vi "Untitled 4.vi"() -> ()   [LabVIEW 2021]
uses:
  <vilib>/userDefined/High Color/IMAQdx.ctl
  <vilib>/MakerHub/LINX/Public/Utilities/Open Serial.vi
  <vilib>/MakerHub/LINX/Public/Sensors/Motion/Servo/Servo Open One Channel.vi
  <vilib>/MakerHub/LINX/Public/Sensors/Motion/Servo/Servo Set Pulse Width One Channel.vi
  <vilib>/MakerHub/LINX/Public/Sensors/Motion/Servo/Servo Close One Channel.vi
  <vilib>/MakerHub/LINX/LMH-LINX.lvlib
  <vilib>/MakerHub/LINX/Public/Sensors/Motion/Servo/Servo.lvlib
  <vilib>/vision/driver/NI_Vision_Acquisition_Software.lvlib
  <vilib>/vision/NI_Vision_Development_Module.lvlib
panel:
  out "Red":bool
  out "Blue":bool
  out "Green":bool
  out "Color Spectrum":dbl[](array[numeric]) format="%.2f"
  out "Image":T1(plugin-control)
  in  "x .or. y?":bool
  out "Error Out":errorcluster
  in  "Serial Port":refnum<visa-resource-name>="N/A"
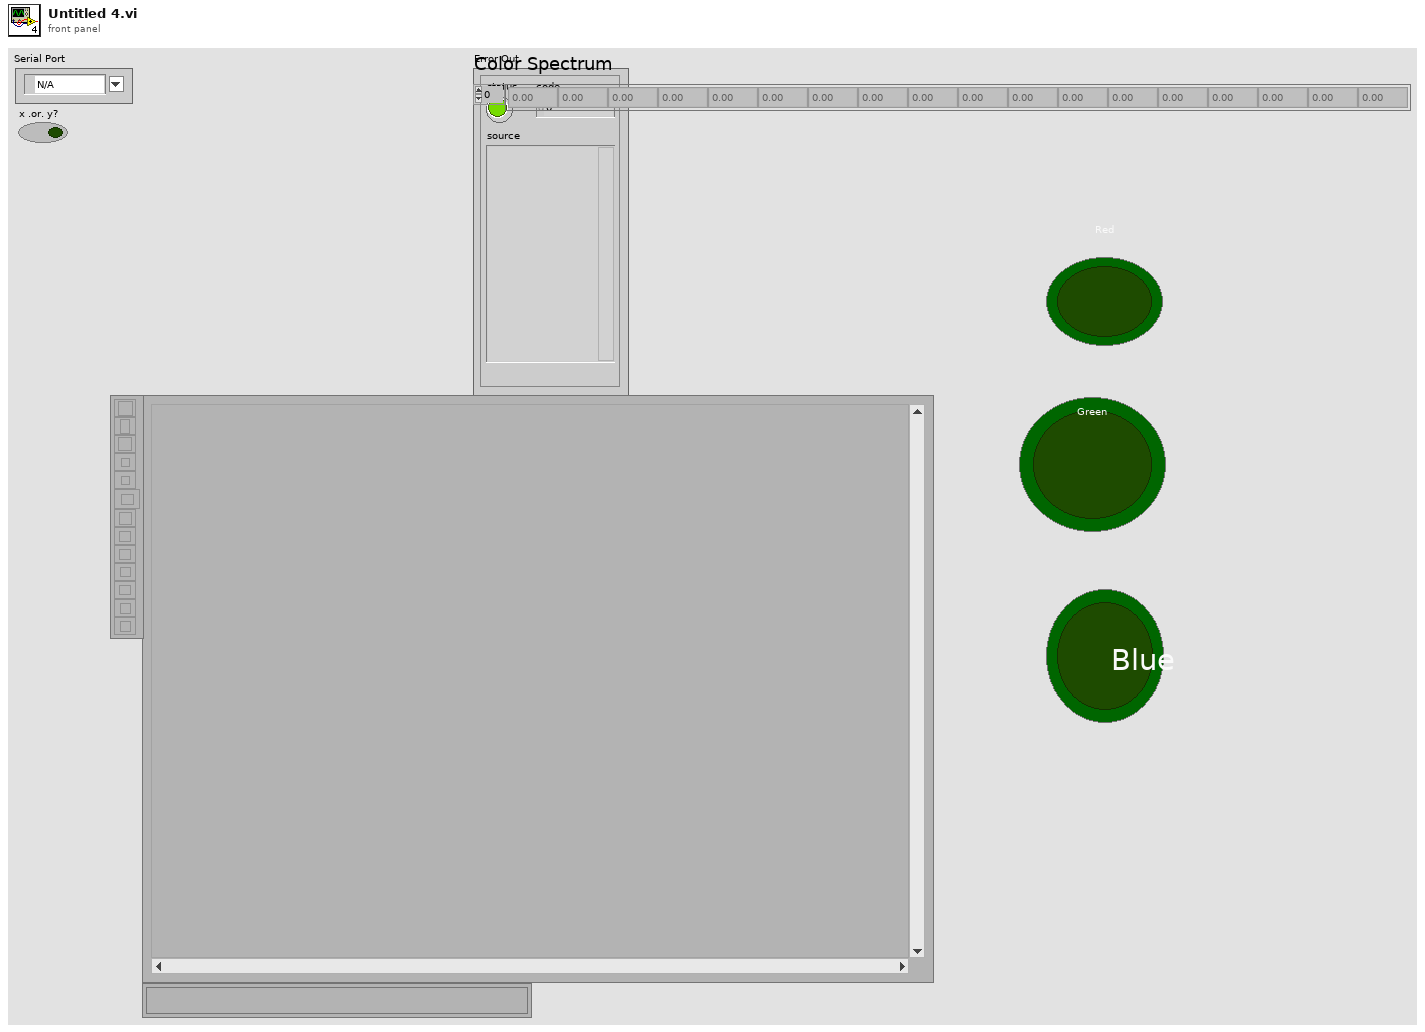
[diagram p1: front panel]
types:
  T1 = typedef "IMAQ Image.ctl" = refnum<image>
  T2 = typedef "IMAQdx.ctl" = refnum<k21>
  T3 = typedef "LMH-LINX.lvlib/LINX Ref.ctl" = cluster{"IO":T4, "Interface":T5, "LINX Device Config":T6}
  T4 = typedef "LMH-LINX.lvlib/Platform.ctl" = enum16{"Remote", "Local"}
  T5 = typedef "LMH-LINX.lvlib/Interface.ctl" = enum16{"Serial", "TCP"}
  T6 = typedef "LMH-LINX.lvlib/Device.lvlib/LINX Device Config.ctl" = cluster{"Interface":T5, "COM Port":refnum<visa-resource-name>, "TCP Configuration":T7, "Device Family":u8, "Device ID":u8, "Device Name":string, "TCP Ref":refnum<k5>, "Channels":T8}
  T7 = typedef "LMH-LINX.lvlib/Device.lvlib/TCP Config.ctl" = cluster{"IP Address":string, "Port":u16}
  T8 = typedef "LMH-LINX.lvlib/Channels.ctl" = cluster{"DI":u8[], "DO":u8[], "AI":u8[], "AO":u8[], "PWM":u8[], "QE":u8[], "UART":u8[], "I2C 2":u8[], "SPI":u8[], "CAN":u8[], "Servo":u8[], "AI Ref (V)":dbl, "AI Resolution (Bits)":u8, "AO Ref (V)":dbl, "AO Resolution (Bits)":u8}
  T9 = cluster{"Global Rectangle":i32[], "Contours":cluster{"Contour Type":u32, "ROI Type":u32, "Points":i32[]}[]}
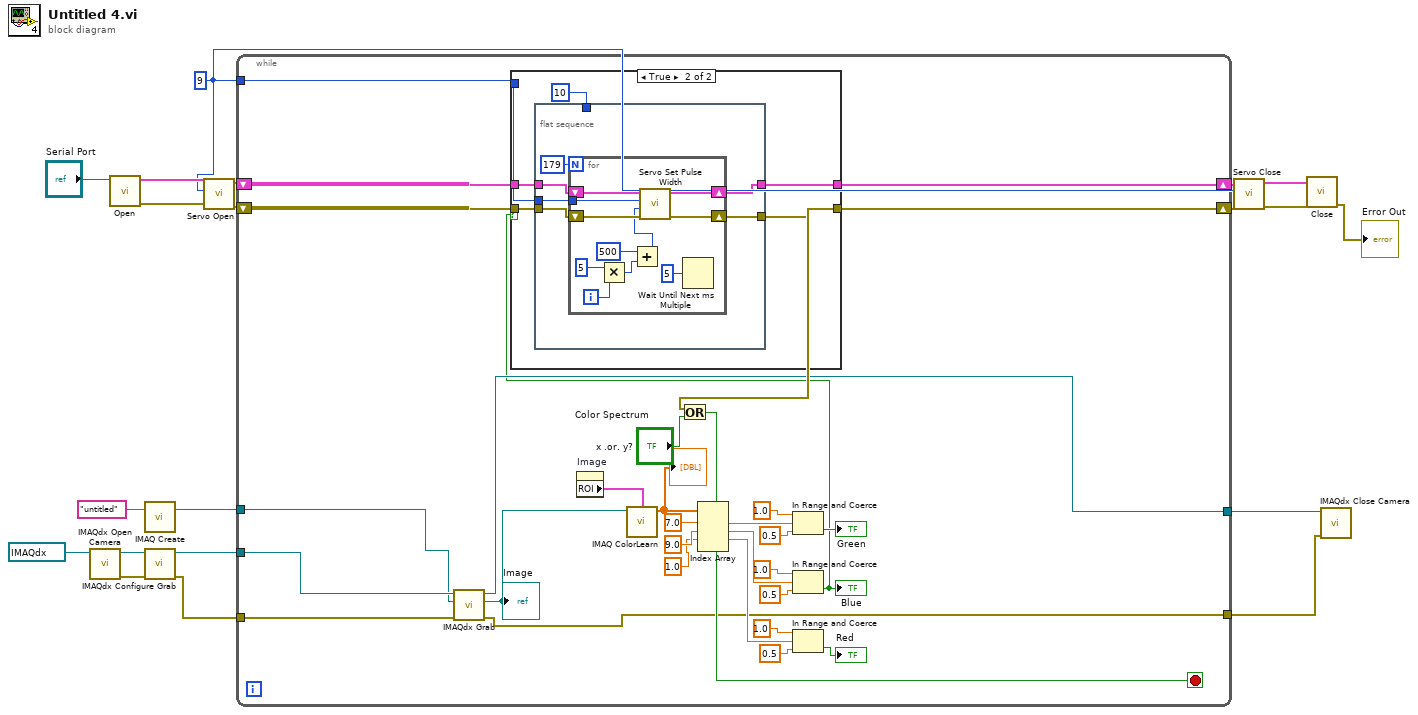
[diagram p0: block diagram]
diagram:
  w10 = u8 9 ("Servo Channel")
  n1 = call <vilib>:"IMAQdx Open Camera.vi"("Session In"=T2 "cam2") -> ("error out"=w9:errorcluster, "Session Out"=w8:T2)  [unwired: 9 in]
  n2 = call-poly <vilib>:"Open.vi"("Serial Port"="Serial Port") -> ("Error Out"=w15:errorcluster, "LINX Resource"=w19:T3)  [unwired: 8 in, 1 out]
  n3 = call "IMAQ Create"("Image Name"="untitled") -> ("New Image"=w3:T1)  [unwired: 4 in, 1 out]
  n4 = call <vilib>:"IMAQdx Configure Grab.vi"("error in"=w9, "Session In"=w8) -> ("error out"=w4:errorcluster, "Session Out"=w5:T2)  [unwired: 8 in]
  n5 = call-poly <vilib>:"Servo Open.vi"("Error In"=w15, "Servo Channel"=w10, "LINX Resource"=w19) -> ("Error Out"=w14:errorcluster, "LINX Resource"=w18:T3)  [unwired: 7 in]
  n6 = while {
    shift-right: [w49] -> w17
    shift-left: w18 -> [w50]
    shift-right: [w45] -> w13
    shift-left: w14 -> [w48]
    tunnel: w10 -> [w47]
    tunnel: w5 -> [w28]
    tunnel: w4 -> [w27]
    tunnel: w3 -> [w26]
    tunnel: [w25] -> w2
    tunnel: [w24] -> w1
    stop <- w46 stop-if-true
    n7 = call <vilib>:"IMAQdx Grab.vi"("error in"=w27, "Image In"=w26, "Session In"=w28) -> ("error out"=w24:errorcluster, "Image Out"=w37:T1, "Session Out"=w25:T2)  [unwired: 5 in, 1 out]
    "Image" <- w37
    n8 = property on="Image" class="ImageControl"() -> ("ROI"=w38:T9)  [unwired: 2 in, 2 out]
    n9 = call "IMAQ ColorLearn"("ROI Descriptor"=w38, "Image"=w37) -> ("Color Spectrum"=w39:dbl[])  [unwired: 6 in, 1 out]
    "Color Spectrum" <- w39
    n10 = Index Array(array=w39, index #1=7.0 ("Numeric"), index #2=9.0 ("Numeric"), index #3=1.0 ("Numeric")) -> (element #1=w40:dbl, element #2=w41:dbl, element #3=w42:dbl)  [unwired: 1 in, 1 out]
    n11 = In Range and Coerce(upper limit=1.0, x=w40, lower limit=0.5) -> (In Range?=→"Green":bool)  [unwired: 1 out]
    n12 = In Range and Coerce(upper limit=1.0, x=w41, lower limit=0.5) -> (In Range?=w23:bool)  [unwired: 1 out]
    "Blue" <- w23
    n13 = case shown="True" w23 {
      tunnel: w50 -> [w52 w58]
      tunnel: [w52 w57] -> w49
      tunnel: w48 -> [w51 w56]
      tunnel: w47 -> [_ w55]
      tunnel: [w51 w54] -> w45
      frame False {
      }
      frame True {
        n14 = flat-sequence {
          tunnel: w58 -> [w64]
          tunnel: [w63] -> w57
          tunnel: w56 -> [w62]
          tunnel: w55 -> [w61]
          tunnel: [w60] -> w54
          tunnel: u32 10 ("millisecond multiple") -> [_]
          frame #0 {
            n15 = for {
              N: 179 -> [_]
              tunnel: w61 -> [w72]
              shift-right: [w74] -> w63
              shift-left: w64 -> [w75]
              shift-right: [w71] -> w60
              shift-left: w62 -> [w73]
              i -> [w69]
              n16 = Multiply(x=5, y=w69) -> (x*y=w67:i32)
              n17 = Add(x=500, y=w67) -> (x+y=w65:i32)
              n18 = call-poly <vilib>:"Servo Set Pulse Width.vi"("Error In"=w73, "Pulse Width (uS)"=w65, "Servo Channel"=w72, "LINX Resource"=w75) -> ("Error Out"=w71:errorcluster, "LINX Resource"=w74:T3)  [unwired: 6 in]
              n19 = Wait Until Next ms Multiple(millisecond multiple=u32 5) -> ()  [unwired: 1 out]
            }
          }
        }
      }
    }
    n20 = Or(x=w45, y="x .or. y?") -> (x .or. y?=w46:bool)
    n21 = In Range and Coerce(upper limit=1.0, x=w42, lower limit=0.5) -> (In Range?=→"Red":bool)  [unwired: 1 out]
  }
  n22 = call-poly <vilib>:"Servo Close.vi"("Error In"=w13, "Servo Channel"=w10, "LINX Resource"=w17) -> ("Error Out"=w12:errorcluster, "LINX Resource"=w16:T3)  [unwired: 7 in]
  n23 = call <vilib>:"Close.vi"("Error In"=w12, "LINX Resource"=w16) -> ("Error Out"=→"Error Out":errorcluster)  [unwired: 9 in]
  n24 = call <vilib>:"IMAQdx Close Camera.vi"("error in"=w1, "Session In"=w2) -> ()  [unwired: 9 in, 1 out]
